vi "Read processing results.vi"(8 "error in":errorcluster, 11 "Shared Memory runtime in":refnum<class "Shared Memory runtime.lvclass">) -> (0 "error out":errorcluster, 2 "processing results":T1[](array[typedef]), 3 "Shared Memory runtime out":refnum<class "Shared Memory runtime.lvclass">)   [LabVIEW 2014, in "Shared Memory runtime.lvclass"]
uses:
  Shared Memory runtime.lvclass
  channel runtime.ctl
  <vilib>/NI/Tag Bus Module Framework/channel/channel classification.ctl
  <vilib>/NI/Tag Bus/tag/Data Type.ctl
  <vilib>/NI/NI Linux RT IPC/Shared Memory/Classes/Shared Memory/Public/Controls/reference.ctl
  <vilib>/NI/NI Linux RT IPC/Shared Memory/Classes/Shared Memory/Shared Memory.lvclass
  Shared Memory runtime.lvclass/Shared Memory runtime.ctl
  <vilib>/NI/Tag Bus Module Framework/channel/TBM channel.lvclass
  <vilib>/NI/Tag Bus/tag/tag descriptor.lvclass
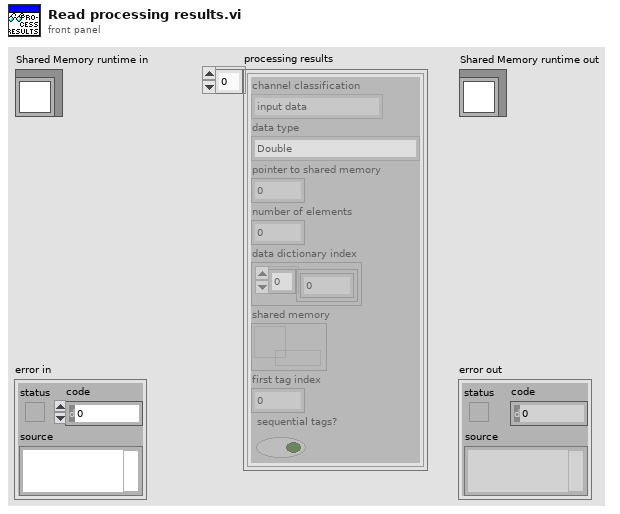
[diagram p1: front panel]
types:
  T1 = typedef "Shared Memory runtime.lvclass/channel runtime.ctl" = cluster{"channel classification":T2, "data type":T3, "pointer to shared memory":u64, "number of elements":u64, "data dictionary index":cluster{i32[]}, "shared memory":T4, "first tag index":i32, "sequential tags?":bool}
  T2 = typedef "TBM channel.lvclass/channel classification.ctl" = enum16{"input data", "output data", "processing parameter", "processing result"}
  T3 = typedef "tag bus.lvlib/tag descriptor.lvclass/Data Type.ctl" = enum16{"Double", "Single", "I64", "I32", "I16", "I8", "U64", "U32", "U16", "U8", "Boolean", "String", "Array of Double", "Array of Single", "Array of I64", "Array of I32", "Array of I16", "Array of I8", "Array of U64", "Array of U32", "Array of U16", "Array of U8", "Array of Boolean", "Array of String"}
  T4 = typedef "Shared Memory.lvlib/Shared Memory.lvclass/reference.ctl" = refnum<data-value>
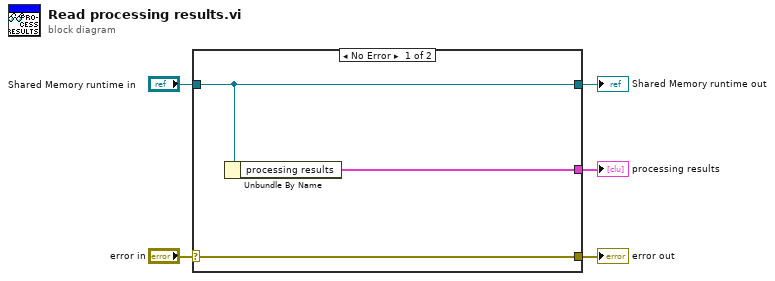
[diagram p0: block diagram]
diagram:
  n1 = case shown="No Error" "error in" {
    selector: "error in" -> [w8 w9]
    tunnel: [w8 w9] -> w4
    tunnel: [w7 w10] -> w2
    tunnel: "Shared Memory runtime in" -> [w7 w10]
    tunnel: [w6 _] -> w1
    frame No Error {
      n2 = Unbundle By Name(w7) -> ("processing results"=w6:T1[])
    }
    frame Error {
    }
  }
  "error out" <- w4
  "Shared Memory runtime out" <- w2
  "processing results" <- w1
